vi "test_serial.vi"(1 "Color Box":u32(colorbox), 2 "VISA resource name":refnum<visa-resource-name>) -> (0 "read buffer":string)   [LabVIEW 2014]
uses:
  <vilib>/Instr/_visa.llb/VISA Configure Serial Port (Instr).vi
panel:
  out "to Send":u8[](array[numeric]) format="%02x"
  out "checksum":u8 format="%02x"
  out "length":u8
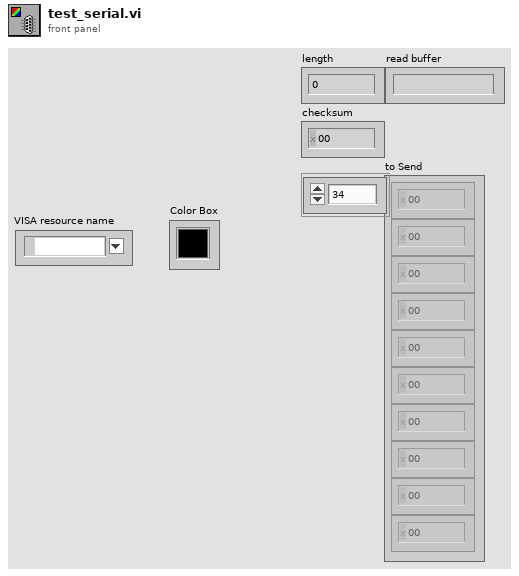
[diagram p1: front panel]
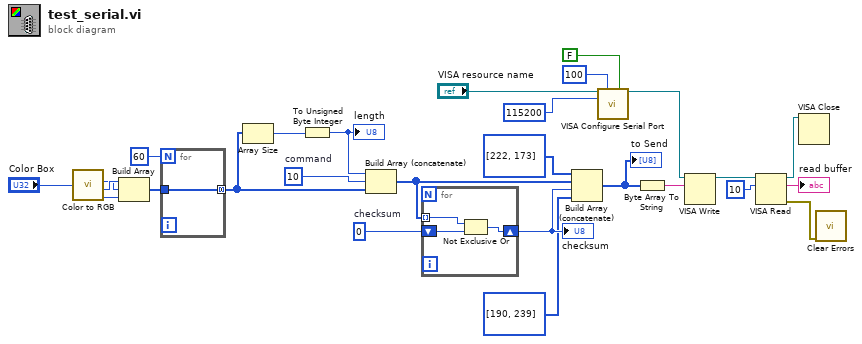
[diagram p0: block diagram]
diagram:
  w19 = u8 10  # command
  w16 = u8 0  # checksum
  n1 = call <vilib>:"Color to RGB.vi"("Color"="Color Box") -> ("R"=w24:u8, "G"=w25:u8, "B"=w23:u8)  [unwired: 1 out]
  n2 = Build Array(w25, w24, w23) -> (w22:u8[])
  n3 = for {
    N: 60 -> [_]
    tunnel: w22 -> [w28]
    tunnel: [w28] -> w18 mode=concatenating
  }
  n4 = Array Size(array=w18) -> (size(s)=w20:i32)
  n5 = To Unsigned Byte Integer(number=w20) -> (unsigned 8bit integer=w17:u8)
  "length" <- w17
  n6 = Build Array (concatenate)(w17, w19, w18) -> (w15:u8[])
  n7 = for {
    tunnel: w15 -> [w31] mode=indexing
    shift-right: [w29] -> w14
    shift-left: w16 -> [w30]
    n8 = Not Exclusive Or(1:w30, 2:w31) -> (0:w29:u8)
  }
  "checksum" <- w14
  n9 = Build Array (concatenate)(u8[] [222, 173], w15, w14, u8[] [190, 239]) -> (w6:u8[])
  "to Send" <- w6
  n10 = call-poly "VISA Configure Serial Port"("VISA resource name"="VISA resource name", "timeout (10sec)"=u32 100, "Enable Termination\nChar (T)"=FALSE ("Enable Termination\nChar (T)"), "baud rate (9600)"=u32 115200) -> ("VISA resource name out"=w9:refnum<visa-resource-name>)  [unwired: 10 in, 1 out]
  n11 = Byte Array To String(unsigned byte array=w6) -> (string=w7:string)
  n12 = VISA Write(VISA resource name=w9, write buffer=w7) -> (VISA resource name out=w5:refnum<visa-resource-name>)  [unwired: 1 in, 2 out]
  n13 = VISA Read(VISA resource name=w5, byte count=u32 10) -> (VISA resource name out=w2:refnum<visa-resource-name>, read buffer=→"read buffer":string, error out=w1:errorcluster)  [unwired: 1 in, 1 out]
  n14 = VISA Close(VISA resource name=w2) -> ()  [unwired: 1 in, 1 out]
  n15 = call <vilib>:"Clear Errors.vi"("error in (no error)"=w1) -> ()  [unwired: 5 in, 2 out]
